vi "Find One Cycle R2.vi"(11 "data in":i32[][](array[numeric])) -> (1 "n crossings":i32, 3 "data out":i32[][](array[numeric]))   [LabVIEW 2018]
uses:
  <vilib>/Analysis/baseanly.llb/Mean (DBL).vi
  <vilib>/ptbypt/NI_PtbyPt.lvlib
  <vilib>/Analysis/NI_AALBase.lvlib
panel:
  in  "Trigger":enum16{"either", "minus-plus", "plus-minus"}(ring)=enum."plus-minus"
  out "crossing indices":i32[](array[numeric])
  out "Plotting Data":i32[](graph) caption="Waveform Chart - dark"
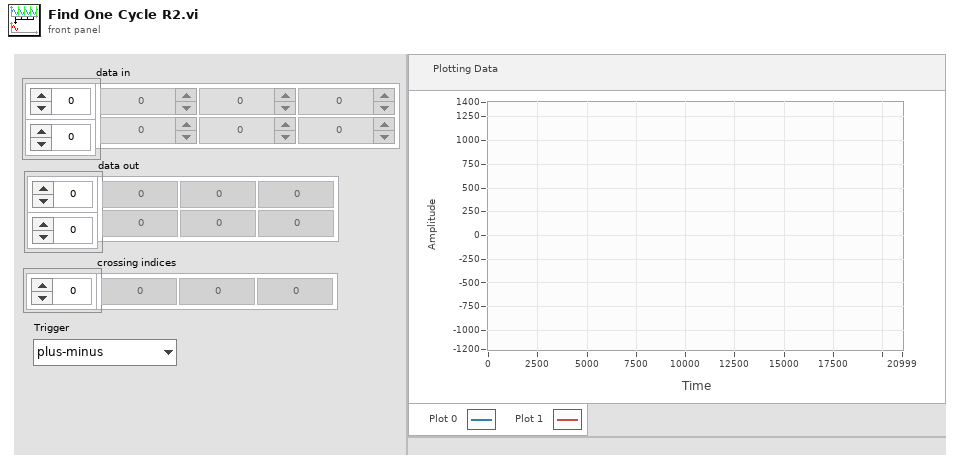
[diagram p1: front panel]
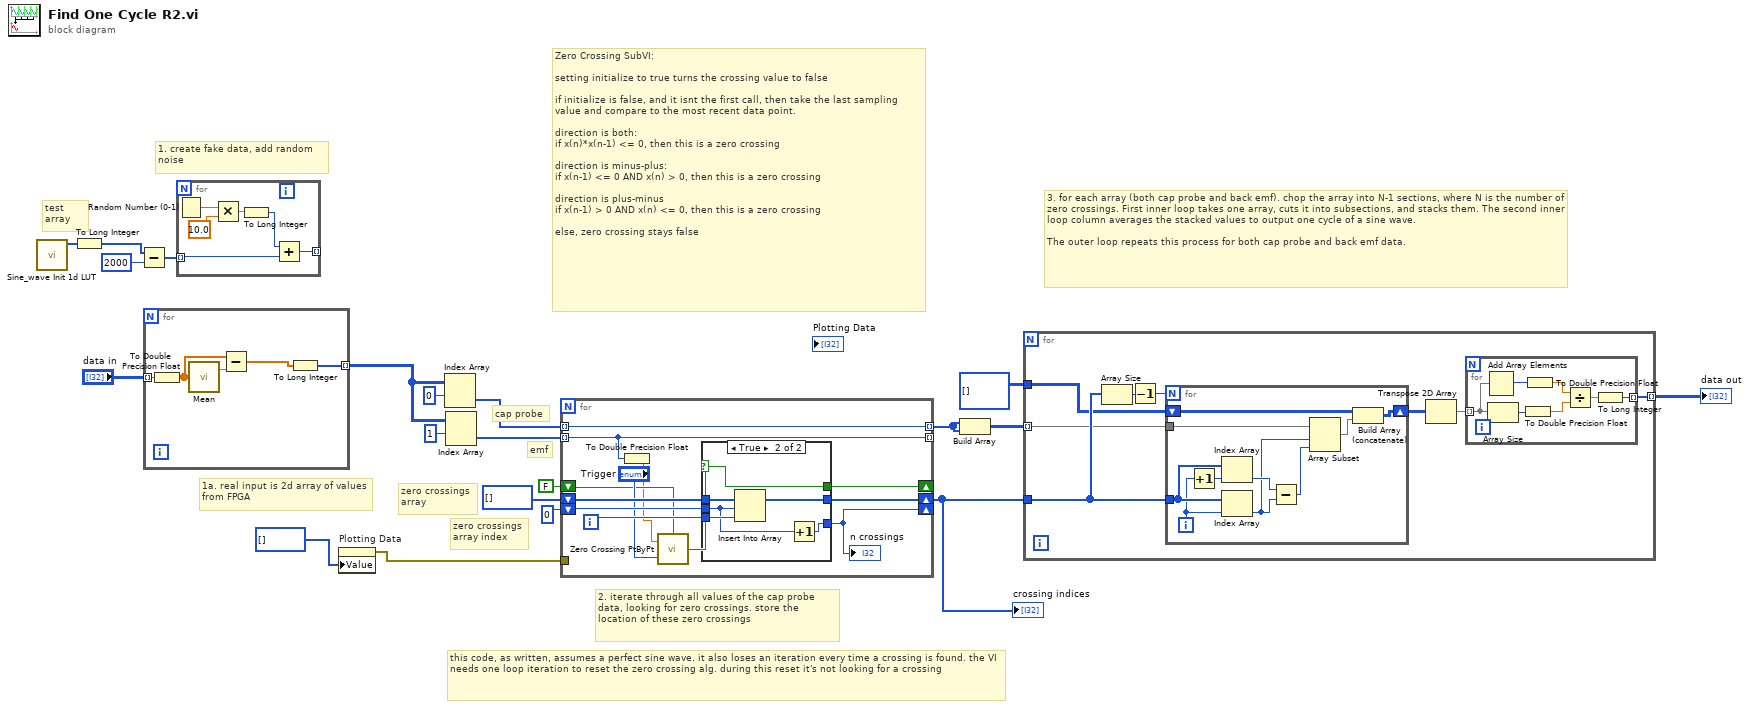
[diagram p0: block diagram]
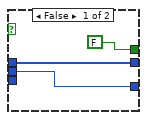
[diagram p2: hidden frame]
diagram:
  # "3. for each array (both cap probe and back emf). chop the array into N-1 sections, where N is the number of zero crossings. First inner loop takes one array, cuts it into subsections, and stacks them. The second inner loop column averages the stacked values to output one cycle of a sine wave.\n\nThe outer loop repeats this process for both cap probe and back emf data."
  # "2. iterate through all values of the cap probe data, looking for zero crossings. store the location of these zero crossings"
  # "1a. real input is 2d array of values from FPGA"
  # "1. create fake data, add random noise"
  # "Zero Crossing SubVI:\n\nsetting initialize to true turns the crossing value to false\n\nif initialize is false, and it isnt the first call, then take the last sampling value and compare to the most recent data point.\n\ndirection is both:\nif x(n)*x(n-1) <= 0, then this is a zero crossing\n\ndirection is minus-plus:\nif x(n-1) <= 0 AND x(n) > 0, then this is a zero crossing\n\ndirection is plus-minus\nif x(n-1) > 0 AND x(n) <= 0, then this is a zero crossing\n\nelse, zero crossing stays false"
  # "test\narray"
  # "cap probe"
  # "emf"
  # "zero crossings\narray index"
  # "zero crossings\narray"
  # "this code, as written, assumes a perfect sine wave. it also loses an iteration every time a crossing is found. the VI needs one loop iteration to reset the zero crossing alg. during this reset it's not looking for a crossing"
  n1 = call "Sine_wave Init 1d LUT.vi"() -> ("Init Data Out"=w12:u16[])  [unwired: 11 in]
  n2 = To Long Integer(number=w12) -> (32bit integer=w11:i32[])
  n3 = Subtract(x=w11, y=2000 ("index (row)")) -> (x-y=w10:i32[])
  n4 = for {
    tunnel: "data in" -> [w24] mode=indexing
    tunnel: [w21] -> w1 mode=indexing
    n5 = To Double Precision Float(number=w24) -> (double precision float=w23:dbl[])
    n6 = call-poly <vilib>:"Mean.vi"("X"=w23) -> ("mean"=w25:dbl)  [unwired: 1 out]
    n7 = Subtract(x=w23, y=w25) -> (x-y=w22:dbl[])
    n8 = To Long Integer(number=w22) -> (32bit integer=w21:i32[])
  }
  n9 = for {
    tunnel: w10 -> [w27] mode=indexing
    tunnel: [w26] -> _ mode=indexing
    n10 = Random Number (0-1)() -> (number: 0 to 1=w31:dbl)
    n11 = Multiply(x=w31, y=10.0 ("index (row)")) -> (x*y=w29:dbl)
    n12 = To Long Integer(number=w29) -> (32bit integer=w28:i32)
    n13 = Add(x=w28, y=w27) -> (x+y=w26:i32)
  }
  n14 = property on="Plotting Data" class="WFChart (strict)"("Value"=i32[] []) -> (error out=w8:errorcluster)  [unwired: 2 in, 1 out]
  n15 = Index Array(array=w1, index (row)=0) -> (element=w3:i32[])  [unwired: 1 in]
  n16 = Index Array(array=w1, index (row)=1) -> (element=w4:i32[])  [unwired: 1 in]
  n17 = for {
    shift-right: [w43] -> w14
    shift-left: i32[] [] ("subarray") -> [w41]
    shift-right: [w38] -> _
    shift-left: 0 ("n cycles") -> [w42]
    shift-right: [w39] -> _
    shift-left: FALSE -> [w34]
    tunnel: w3 -> [w40] mode=indexing
    tunnel: [w40] -> w13 mode=indexing
    tunnel: w4 -> [w36] mode=indexing
    tunnel: [w36] -> _ mode=indexing
    tunnel: w8 -> [_]
    i -> [w37]
    n18 = To Double Precision Float(number=w36) -> (double precision float=w32:dbl)
    n19 = call <vilib>:"Zero Crossing PtByPt.vi"("initialize"=w34, "direction"="Trigger", "input data point"=w32) -> ("crossing"=w33:bool)
    n20 = case shown="True" w33 {
      selector: w33 -> [_ w49]
      tunnel: [w46 w52] -> w38
      tunnel: [w45 w50] -> w43
      tunnel: w42 -> [w46 w47]
      tunnel: w41 -> [w45 w51]
      tunnel: [FALSE w49] -> w39
      tunnel: w37 -> [_ w48]
      frame False {
      }
      frame True {
        n21 = Insert Into Array(array=w51, index=w47, new element=w48) -> (w50:i32[])
        n22 = Increment(x=w47) -> (x+1=w52:i32)
      }
    }
    "n crossings" <- w38
  }
  "crossing indices" <- w14
  n23 = Build Array(w13, w13) -> (w6:i32[][])
  n24 = for {
    tunnel: w14 -> [w60]
    tunnel: i32[][] [] -> [w59]
    tunnel: w6 -> [w56] mode=indexing
    tunnel: [w53] -> w5 mode=indexing
    n25 = Array Size(array=w60) -> (size(s)=w58:i32)
    n26 = Decrement(x=w58) -> (x-1=w57:i32)
    n27 = for {
      N: w57 -> [_]
      tunnel: w56 -> [w77]
      shift-right: [w68] -> w54
      shift-left: w59 -> [w69]
      tunnel: w60 -> [w76]
      i -> [w75]
      n28 = Increment(x=w75) -> (x+1=w74:i32)
      n29 = Index Array(array=w76, index=w74) -> (element=w72:i32)
      n30 = Index Array(array=w76, index=w75) -> (element=w71:i32)
      n31 = Subtract(x=w72, y=w71) -> (x-y=w73:i32)
      n32 = Array Subset(array=w77, index=w71, length=w73) -> (w70:i32[])
      n33 = Build Array (concatenate)(w69, w70) -> (w68:i32[][])
    }
    n34 = Transpose 2D Array(2D array=w54) -> (transposed array=w55:i32[][])
    n35 = for {
      tunnel: w55 -> [w67] mode=indexing
      tunnel: [w61] -> w53 mode=indexing
      n36 = Add Array Elements(numeric array=w67) -> (sum=w66:i32)
      n37 = Array Size(array=w67) -> (size(s)=w65:i32)
      n38 = To Double Precision Float(number=w65) -> (double precision float=w64:dbl)
      n39 = To Double Precision Float(number=w66) -> (double precision float=w63:dbl)
      n40 = Divide(x=w63, y=w64) -> (x/y=w62:dbl)
      n41 = To Long Integer(number=w62) -> (32bit integer=w61:i32)
    }
  }
  "data out" <- w5
